vi "Quit Actors.vi"(8 "error in (no error)":errorcluster, 10 "Actor":T1(ring), 11 "Main.lvlib:Main.lvclass":refnum<class "Main.lvclass">) -> (0 "error out":errorcluster, 3 "Main.lvlib:Main.lvclass 2":refnum<class "Main.lvclass">)   [LabVIEW 2018, in "Main.lvlib" / "Main.lvclass"]
uses:
  Main.lvclass
  Main.lvclass/Main.ctl
  <vilib>/ActorFramework/Message Enqueuer/Message Enqueuer.lvclass/Message Enqueuer.ctl
  <vilib>/ActorFramework/Message Enqueuer/Enqueue.vi
  <vilib>/ActorFramework/Stop Msg/Stop Msg.lvclass
  C:/Program Files/National Instruments/LabVIEW 2018/vi.lib/ActorFramework/Message/Message.lvclass
  <vilib>/ActorFramework/Message Priority Queue/Priority Enqueue.vi
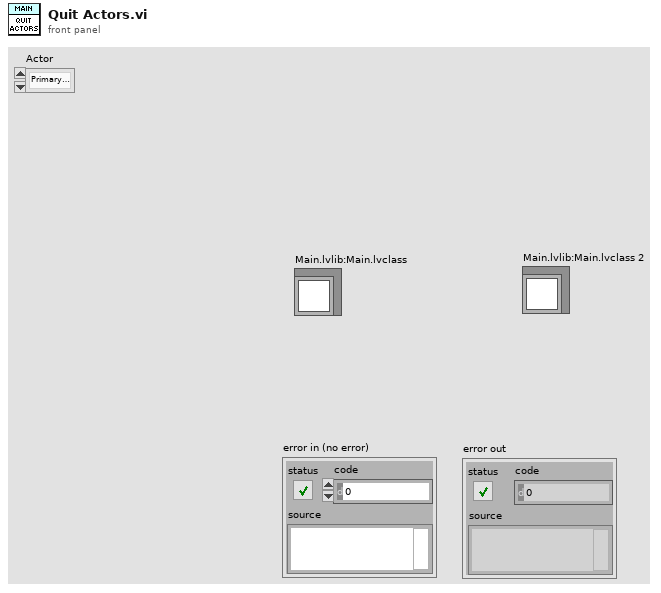
[diagram p1: front panel]
types:
  T1 = enum16{"Primary Feeder", "Chamber Pressure", "Feeder Pressure", "Stage", "Outer MFC", "Inner MFC", "Secondary Feeder", "All"}
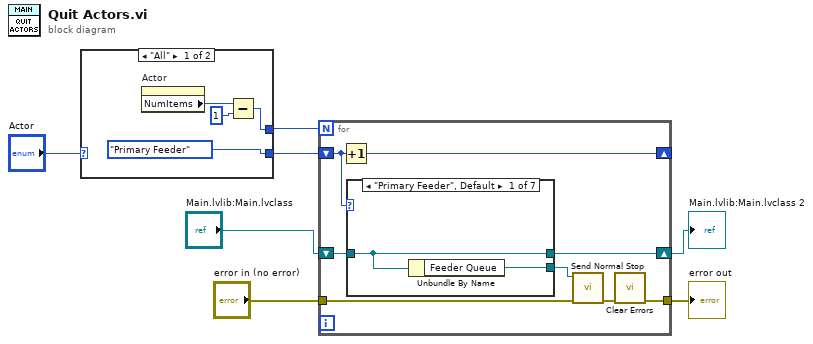
[diagram p0: block diagram]
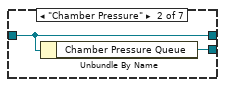
[diagram p2: hidden frame]
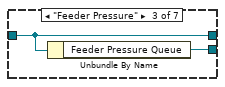
[diagram p3: hidden frame]
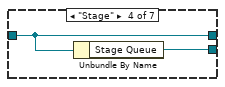
[diagram p4: hidden frame]
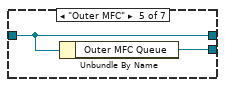
[diagram p5: hidden frame]
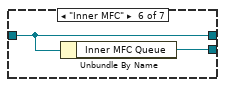
[diagram p6: hidden frame]
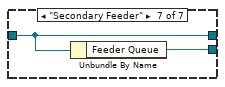
[diagram p7: hidden frame]
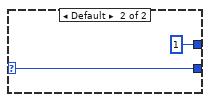
[diagram p8: hidden frame]
diagram:
  n1 = case shown="\"All\"" "Actor" {
    selector: "Actor" -> [_ w12]
    tunnel: [w11 1] -> w5
    tunnel: [T1."Primary Feeder" ("Actor 2") w12] -> w6
    frame "All" {
      n2 = property on="Actor" class="Enum (strict)"() -> ("NumItems"=w10:u32)  [unwired: 2 in, 2 out]
      n3 = Subtract(x=w10, y=u32 1) -> (x-y=w11:u32)
    }
    frame Default {
    }
  }
  n4 = for {
    N: w5 -> [_]
    shift-right: [w21] -> _
    shift-left: w6 -> [w20]
    shift-right: [w17] -> w7
    shift-left: "Main.lvlib:Main.lvclass" -> [w19]
    tunnel: "error in (no error)" -> [w18]
    tunnel: [w14] -> w2
    n5 = Increment(x=w20) -> (x+1=w21:T1)
    n6 = case shown="\"Primary Feeder\", Default" w20 {
      tunnel: w19 -> [w22 w24 w26 w28 w31 w32 w34]
      tunnel: [w22 w24 w26 w28 w31 w32 w34] -> w17
      tunnel: [w23 w25 w27 w29 w30 w33 w35] -> w15
      frame "Primary Feeder", Default {
        n7 = Unbundle By Name(w22) -> ("Feeder Queue"=w23:refnum<class "Message Enqueuer.lvclass">)
      }
      frame "Chamber Pressure" {
        n8 = Unbundle By Name(w24) -> ("Chamber Pressure Queue"=w25:refnum<class "Message Enqueuer.lvclass">)
      }
      frame "Feeder Pressure" {
        n9 = Unbundle By Name(w26) -> ("Feeder Pressure Queue"=w27:refnum<class "Message Enqueuer.lvclass">)
      }
      frame "Stage" {
        n10 = Unbundle By Name(w28) -> ("Stage Queue"=w29:refnum<class "Message Enqueuer.lvclass">)
      }
      frame "Outer MFC" {
        n11 = Unbundle By Name(w31) -> ("Outer MFC Queue"=w30:refnum<class "Message Enqueuer.lvclass">)
      }
      frame "Inner MFC" {
        n12 = Unbundle By Name(w32) -> ("Inner MFC Queue"=w33:refnum<class "Message Enqueuer.lvclass">)
      }
      frame "Secondary Feeder" {
        n13 = Unbundle By Name(w34) -> ("Feeder Queue"=w35:refnum<class "Message Enqueuer.lvclass">)
      }
    }
    n14 = call <vilib>:"Send Normal Stop.vi"("error in (no error)"=w18, "Message Enqueuer"=w15) -> ("error out"=w16:errorcluster)  [unwired: 9 in]
    n15 = call <vilib>:"Clear Errors.vi"("error in (no error)"=w16) -> ("error out"=w14:errorcluster)  [unwired: 5 in, 1 out]
  }
  "error out" <- w2
  "Main.lvlib:Main.lvclass 2" <- w7
